vi "练习一：控制信号发生器开关.vi"   [LabVIEW 2021]
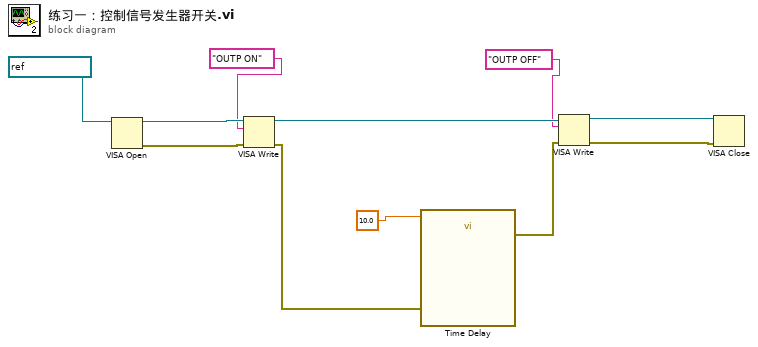
[diagram p0: block diagram]
diagram:
  n1 = VISA Open(VISA resource name=refnum<visa-resource-name> "DG1022U") -> (VISA resource name=w6:refnum<visa-resource-name>, error out=w11:errorcluster)  [unwired: 4 in]
  n2 = VISA Write(VISA resource name=w6, write buffer="OUTP ON", error in (no error)=w11) -> (VISA resource name out=w5:refnum<visa-resource-name>, error out=w9:errorcluster)  [unwired: 1 out]
  n3 = call "Time Delay"("error in (no error)"=w9, "Delay Time (s)"=10.0) -> ("error out"=w8:errorcluster)  [unwired: 9 in]
  n4 = VISA Write(VISA resource name=w5, write buffer="OUTP OFF", error in (no error)=w8) -> (VISA resource name out=w4:refnum<visa-resource-name>, error out=w7:errorcluster)  [unwired: 1 out]
  n5 = VISA Close(VISA resource name=w4, error in (no error)=w7) -> ()  [unwired: 1 out]
